vi "Multiply_IQ.vi"(6 "Sin":fxp<+/-,16,0>, 7 "Cos":fxp<+/-,16,0>, 8 "input valid":bool=TRUE, 10 "Q":fxp<+/-,16,14>, 11 "I":fxp<+/-,16,14>) -> (0 "output valid":bool, 3 "Z":i16)   [LabVIEW 2013]
uses:
  <vilib>/rvi/FXPMathLib/FxpConvert/subVIs/nifxpmath_Convert_SimConfig.ctl
  <vilib>/fxp/LVFixedPointQuantizationPolicyTypeDef.ctl
  <vilib>/fxp/LVFixedPointOverflowPolicyTypeDef.ctl
  <vilib>/rvi/FXPMathLib/FxpConvert/simVIs/DllFxpConvertTemp_sub.vi
  <vilib>/rvi/FXPMathLib/FxpConvert/XNode/nifxpmath_Convert.xnode
  <vilib>/rvi/FXPMathLib/FxpSub/XNode/nifxpmath_Sub.xnode
  <vilib>/rvi/FXPMathLib/FxpMul/XNode/nifxpmath_Multiplier.xnode
  <vilib>/rvi/FXPMathLib/sim/FxpSim.dll
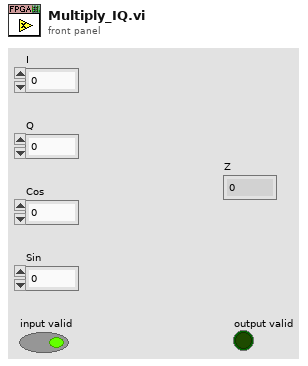
[diagram p1: front panel]
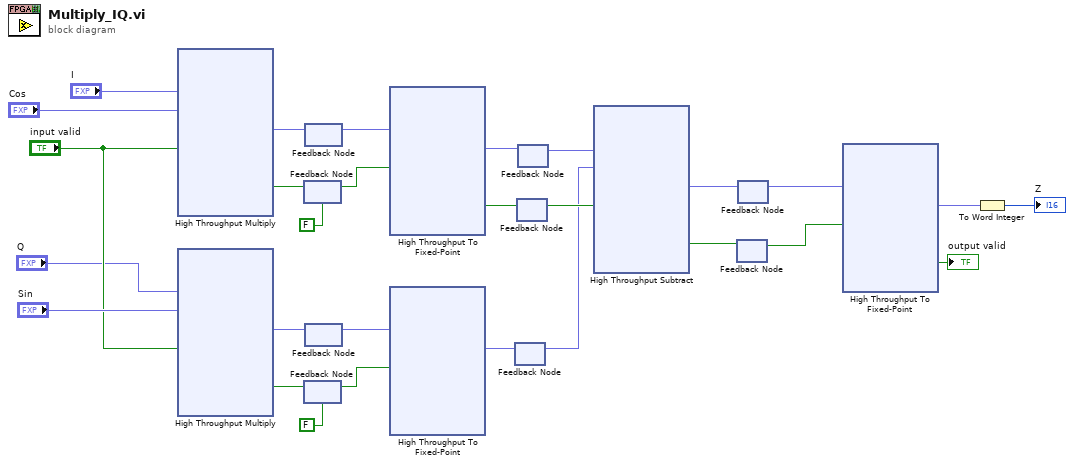
[diagram p0: block diagram]
diagram:
  n1 = xnode "High Throughput Multiply"("x"="I", "y"="Cos", "input valid"="input valid") -> ("x*y"=w28:fxp<+/-,32,14>, "output valid"=w27:bool)  [unwired: 1 in, 1 out]
  n2 = xnode "High Throughput Multiply"("x"="Q", "y"="Sin", "input valid"="input valid") -> ("x*y"=w16:fxp<+/-,32,14>, "output valid"=w15:bool)  [unwired: 1 in, 1 out]
  n3 = feedback #1(FALSE ("output valid")) -> (w20:bool)
  n4 = feedback-in #1(w27) -> ()
  n5 = feedback #2(FALSE ("output valid")) -> (w19:bool)
  n6 = feedback-in #2(w15) -> ()
  n7 = feedback #3() -> (w21:fxp<+/-,32,14>)  [unwired: 1 in]
  n8 = feedback-in #3(w28) -> ()
  n9 = feedback #4() -> (w18:fxp<+/-,32,14>)  [unwired: 1 in]
  n10 = feedback-in #4(w16) -> ()
  n11 = xnode "High Throughput To Fixed-Point"("x"=w21, "input valid"=w20) -> ("y"=w6:fxp<+/-,16,14>, "output valid"=w4:bool)  [unwired: 1 in, 1 out]
  n12 = xnode "High Throughput To Fixed-Point"("x"=w18, "input valid"=w19) -> ("y"=w2:fxp<+/-,16,14>)  [unwired: 1 in, 2 out]
  n13 = feedback #5() -> (w1:fxp<+/-,16,14>)  [unwired: 1 in]
  n14 = feedback-in #5(w2) -> ()
  n15 = feedback #6() -> (w3:bool)  [unwired: 1 in]
  n16 = feedback-in #6(w4) -> ()
  n17 = feedback #7() -> (w5:fxp<+/-,16,14>)  [unwired: 1 in]
  n18 = feedback-in #7(w6) -> ()
  n19 = xnode "High Throughput Subtract"("x"=w5, "y"=w1, "input valid"=w3) -> ("x-y"=w14:fxp<+/-,17,15>, "output valid"=w12:bool)  [unwired: 1 in, 1 out]
  n20 = feedback #8() -> (w11:bool)  [unwired: 1 in]
  n21 = feedback-in #8(w12) -> ()
  n22 = feedback #9() -> (w13:fxp<+/-,17,15>)  [unwired: 1 in]
  n23 = feedback-in #9(w14) -> ()
  n24 = xnode "High Throughput To Fixed-Point"("x"=w13, "input valid"=w11) -> ("y"=w10:fxp<+/-,16,14>, "output valid"=→"output valid":bool)  [unwired: 1 in, 1 out]
  n25 = To Word Integer(number=w10) -> (16bit integer=→"Z":i16)
